vi "behavior_test_no_output.vi"() -> ()   [LabVIEW 2019]
doc: "The myRIO Project template acquires acceleration data from the onboard accelerometer and displays the changes of acceleration values in a waveform chart."
uses:
  <vilib>/myRIO/Common/Instrument Driver Framework/myRIO v1.0/Encoder/typedefs/Encoder Signal Mode.ctl
  <vilib>/myRIO/Instrument Drivers/Onboard IO/Encoder/typedefs/Encoder Reference.ctl
  <vilib>/myRIO/Common/Instrument Driver Framework/Utilities/typedefs/myRIO Generic Hardware Reference.ctl
  <vilib>/myRIO/Common/Instrument Driver Framework/Utilities/typedefs/Hardware Version Enum.ctl
  <vilib>/myRIO/Common/Instrument Driver Framework/Utilities/typedefs/myRIO v1.0 Reference.ctl
  <vilib>/myRIO/Common/Instrument Driver Framework/Utilities/typedefs/Generic FPGA Reference.ctl
  <vilib>/myRIO/Common/Instrument Driver Framework/myRIO v1.0/Encoder/typedefs/Encoder Channels Enum.ctl
  <vilib>/myRIO/Common/Instrument Driver Framework/myRIO v1.0/Encoder/typedefs/Encoder Configuration v1.0.ctl
  <vilib>/userdefined/High Color/nirio_resource_hc.ctl
  <vilib>/myRIO/Instrument Drivers/Onboard IO/DIO/typedefs/DIO Reference.ctl
  <vilib>/myRIO/Common/Instrument Driver Framework/myRIO v1.0/DIO/typedefs/DIO Channels List.ctl
  <vilib>/myRIO/Common/Instrument Driver Framework/myRIO v1.0/DIO/typedefs/DIO Channels Enum.ctl
  <vilib>/myRIO/Common/Instrument Driver Framework/Utilities/vis/Is FPGA Ref Available.vi
  <vilib>/myRIO/Common/Instrument Driver Framework/myRIO v1.0/Encoder/vis/myRIO v1.1 Open Encoder.vi
  <vilib>/myRIO/Instrument Drivers/Onboard IO/Encoder/vis/Read.vi
  <vilib>/myRIO/Common/Instrument Driver Framework/myRIO v1.0/DIO/vis/myRIO v1.1 Open DIO.vi
  <vilib>/myRIO/Instrument Drivers/Onboard IO/DIO/vis/Write.vi
  <vilib>/myRIO/Instrument Drivers/Onboard IO/DIO/vis/Read.vi
  <vilib>/myRIO/Common/Instrument Driver Framework/Utilities/vis/Validate Channels.vi
  <vilib>/myRIO/Common/Instrument Driver Framework/myRIO v1.0/Encoder/vis/myRIO v1.0 Reserve Encoder.vi
  <vilib>/myRIO/Common/Instrument Driver Framework/myRIO v1.0/DIO/vis/myRIO v1.0 Reserve DIO.vi
  <vilib>/myRIO/Common/Instrument Driver Framework/myRIO v1.0/Encoder/vis/myRIO v1.0 Build MUX Configuration Encoder.vi
  <vilib>/myRIO/Common/Instrument Driver Framework/myRIO v1.0/Resource Manager/vis/myRIO v1.0 Reserve Channel List.vi
  <vilib>/myRIO/Common/Instrument Driver Framework/myRIO v1.0/DIO/vis/myRIO v1.0 Build MUX Configuration DIO.vi
  <vilib>/myRIO/Common/Instrument Driver Framework/myRIO v1.0/Resource Manager/vis/myRIO v1.0 Create Configuration List.vi
  <vilib>/myRIO/Common/Instrument Driver Framework/myRIO v1.0/Resource Manager/vis/myRIO v1.0 Reserve Channel.vi
  <vilib>/myRIO/Common/Instrument Driver Framework/myRIO v1.0/Resource Manager/vis/myRIO v1.0 Unreserve Channel.vi
  <vilib>/myRIO/Common/Instrument Driver Framework/myRIO v1.0/Resource Manager/vis/myRIO v1.0 Build Mutex Name.vi
  <vilib>/Utility/VariantDataType/GetNumericInfo.vi
  <vilib>/Utility/error.llb/Error Cluster From Error Code.vi
  <vilib>/myRIO/Common/Instrument Driver Framework/myRIO v1.0/myRIO v1.1 Open.vi
  <vilib>/myRIO/Common/Instrument Driver Framework/Utilities/vis/IO Manager.vi
  <vilib>/myRIO/Common/Instrument Driver Framework/Utilities/vis/Configuration Manager.vi
  <vilib>/myRIO/Common/Instrument Driver Framework/myRIO v1.0/Resource Manager/vis/myRIO v1.0 Configure IO.vi
  <vilib>/myRIO/Common/Instrument Driver Framework/myRIO v1.0/myRIO v1.0 Close.vi
  <vilib>/myRIO/Common/Instrument Driver Framework/myRIO v1.0/Encoder/vis/myRIO v1.0 Configure Encoder.vi
  <vilib>/myRIO/Common/Instrument Driver Framework/myRIO v1.0/Encoder/vis/myRIO v1.0 Read Encoder.vi
  <vilib>/myRIO/Common/Instrument Driver Framework/myRIO v1.0/DIO/vis/myRIO v1.0 Read DIO.vi
  <vilib>/myRIO/Common/Instrument Driver Framework/myRIO v1.0/DIO/vis/myRIO v1.0 Write DIO.vi
  <vilib>/myRIO/Express VI/Onboard IO/Encoder/Encoder Express VI.xnode
  <vilib>/myRIO/Instrument Drivers/Onboard IO/Encoder/vis/myRIO Encoder Open.xnode
  <vilib>/myRIO/Common/Instrument Driver Framework/myRIO v1.0/Encoder/typedefs/Encoder Count Direction Enum.ctl
  <vilib>/myRIO/Express VI/Onboard IO/DI/DI Express VI.xnode
  <vilib>/myRIO/Instrument Drivers/Onboard IO/DIO/vis/myRIO DIO Open.xnode
  <vilib>/myRIO/Express VI/Onboard IO/DO/DO Express VI.xnode
  <vilib>/myRIO/Instrument Drivers/Onboard IO/Encoder/Encoder.lvlib
  <vilib>/myRIO/Instrument Drivers/Onboard IO/DIO/DIO.lvlib
panel:
  out "Reward_mat":dbl[](array[numeric])
  out "Reward":bool=TRUE
  out "Trial":u32
  out "Frame clock":i32
  out "Licks":u32
  out "Lick":bool
  out "Output":dbl[][](array[numeric])
  out "Time":dbl
  out "Overflow?":bool
  out "Counter Value":i32
  out "Velocity":dbl
  out "Velocity Plot":dbl[](graph)
  out "Velocity array":dbl[](array[numeric])
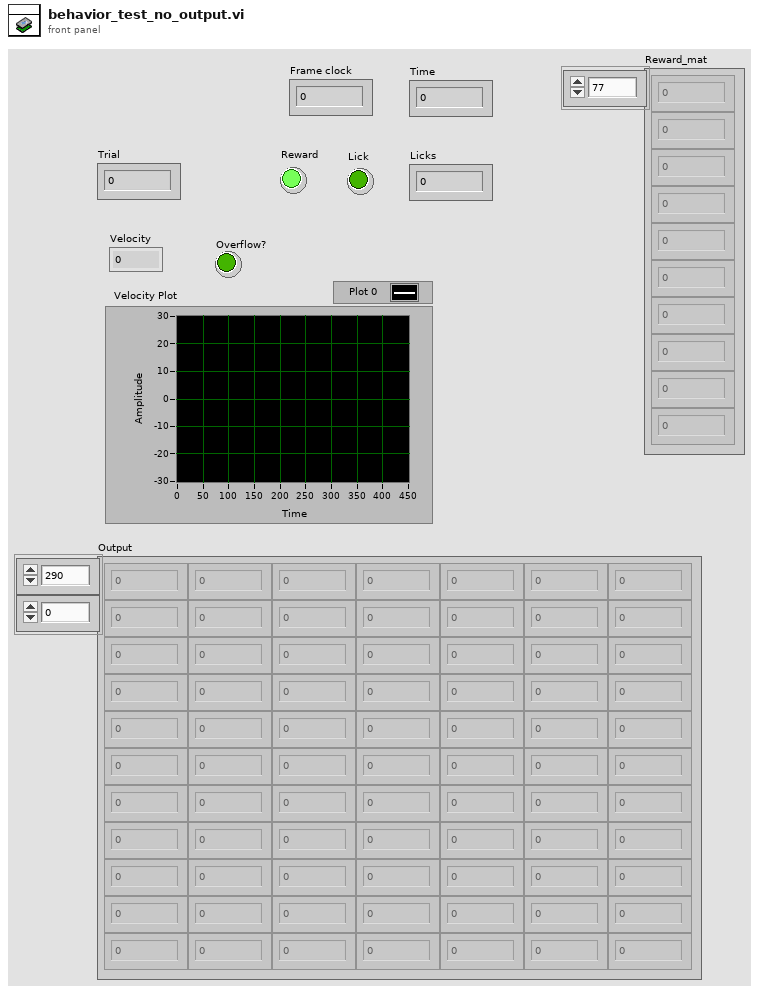
[diagram p1: front panel]
types:
  T1 = typedef "Encoder.lvlib/Encoder Reference.ctl" = cluster{"myRIO Reference":T2, "Encoder Channels Enum":T6}
  T2 = typedef "myRIO Generic Hardware Reference.ctl" = cluster{"myRIO Model":T3, "myRIO Hardware Reference":T4}
  T3 = typedef "Hardware Version Enum.ctl" = enum16{"Unknown", "myRIO-1900", "myRIO-1950", "roboRIO", "NI ELVIS RIO CM", "ELVIS III"}
  T4 = typedef "myRIO v1.0 Reference.ctl" = cluster{"Generic FPGA Reference":T5, "Allow multiple opens":bool}
  T5 = typedef "Generic FPGA Reference.ctl" = refnum<k20>
  T6 = typedef "Encoder Channels Enum.ctl" = enum16{"Not Connected", "C/ENC0", "C/ENC1", "A/ENC", "A/ENC0", "A/ENC1", "A/ENC2", "A/ENC3", "A/ENC4", "A/ENC5", "A/ENC6", "A/ENC7", "A/ENC8", "A/ENC9", "B/ENC", "B/ENC0", "B/ENC1", "B/ENC2", "B/ENC3", "B/ENC4", "B/ENC5", "B/ENC6", "B/ENC7", "B/ENC8", "B/ENC9", "DIO/ENC0", "DIO/ENC1", "DIO/ENC2", "DIO/ENC3", "DIO/ENC4"}
  T7 = typedef "Encoder Signal Mode.ctl" = enum16{"Quadrature phase signal", "Step and direction signal"}
  T8 = typedef "nirio_resource_hc.ctl" = tag
  T9 = typedef "DIO.lvlib/DIO Reference.ctl" = cluster{"myRIO Reference":T2, "DIO Channels List":T10}
  T10 = typedef "DIO Channels List.ctl" = T11[]
  T11 = typedef "DIO Channels Enum.ctl" = enum16{"Not Connected", "C/DIO0", "C/DIO1", "C/DIO2", "C/DIO3", "C/DIO4", "C/DIO5", "C/DIO6", "C/DIO7", "A/DIO0", "A/DIO1", "A/DIO2", "A/DIO3", "A/DIO4", "A/DIO5", "A/DIO6", "A/DIO7", "A/DIO8", "A/DIO9", "A/DIO10", "A/DIO11", "A/DIO12", "A/DIO13", "A/DIO14", "A/DIO15", "A/DIO16", "A/DIO17", "A/DIO18", "A/DIO19", "B/DIO0", "B/DIO1", "B/DIO2", "B/DIO3", "B/DIO4", "B/DIO5", "B/DIO6", "B/DIO7", "B/DIO8", "B/DIO9", "B/DIO10", "B/DIO11", "B/DIO12", "B/DIO13", "B/DIO14", "B/DIO15", "B/DIO16", "B/DIO17", "B/DIO18", "B/DIO19", "LED0", "LED1", "LED2", "LED3", "Button0", "DIO/DIO0", "DIO/DIO1", "DIO/DIO2", "DIO/DIO3", "DIO/DIO4", "DIO/DIO5", "DIO/DIO6", "DIO/DIO7", "DIO/DIO8", "DIO/DIO9", "SPI/CS0", "SPI/CS1", "SPI/CS2", "SPI/CS3", "LED RADIO (Green)", "LED RADIO (Red)", "LED COMM (Green)", "LED COMM (Red)", "LED MODE (Green)", "LED MODE (Red)"}
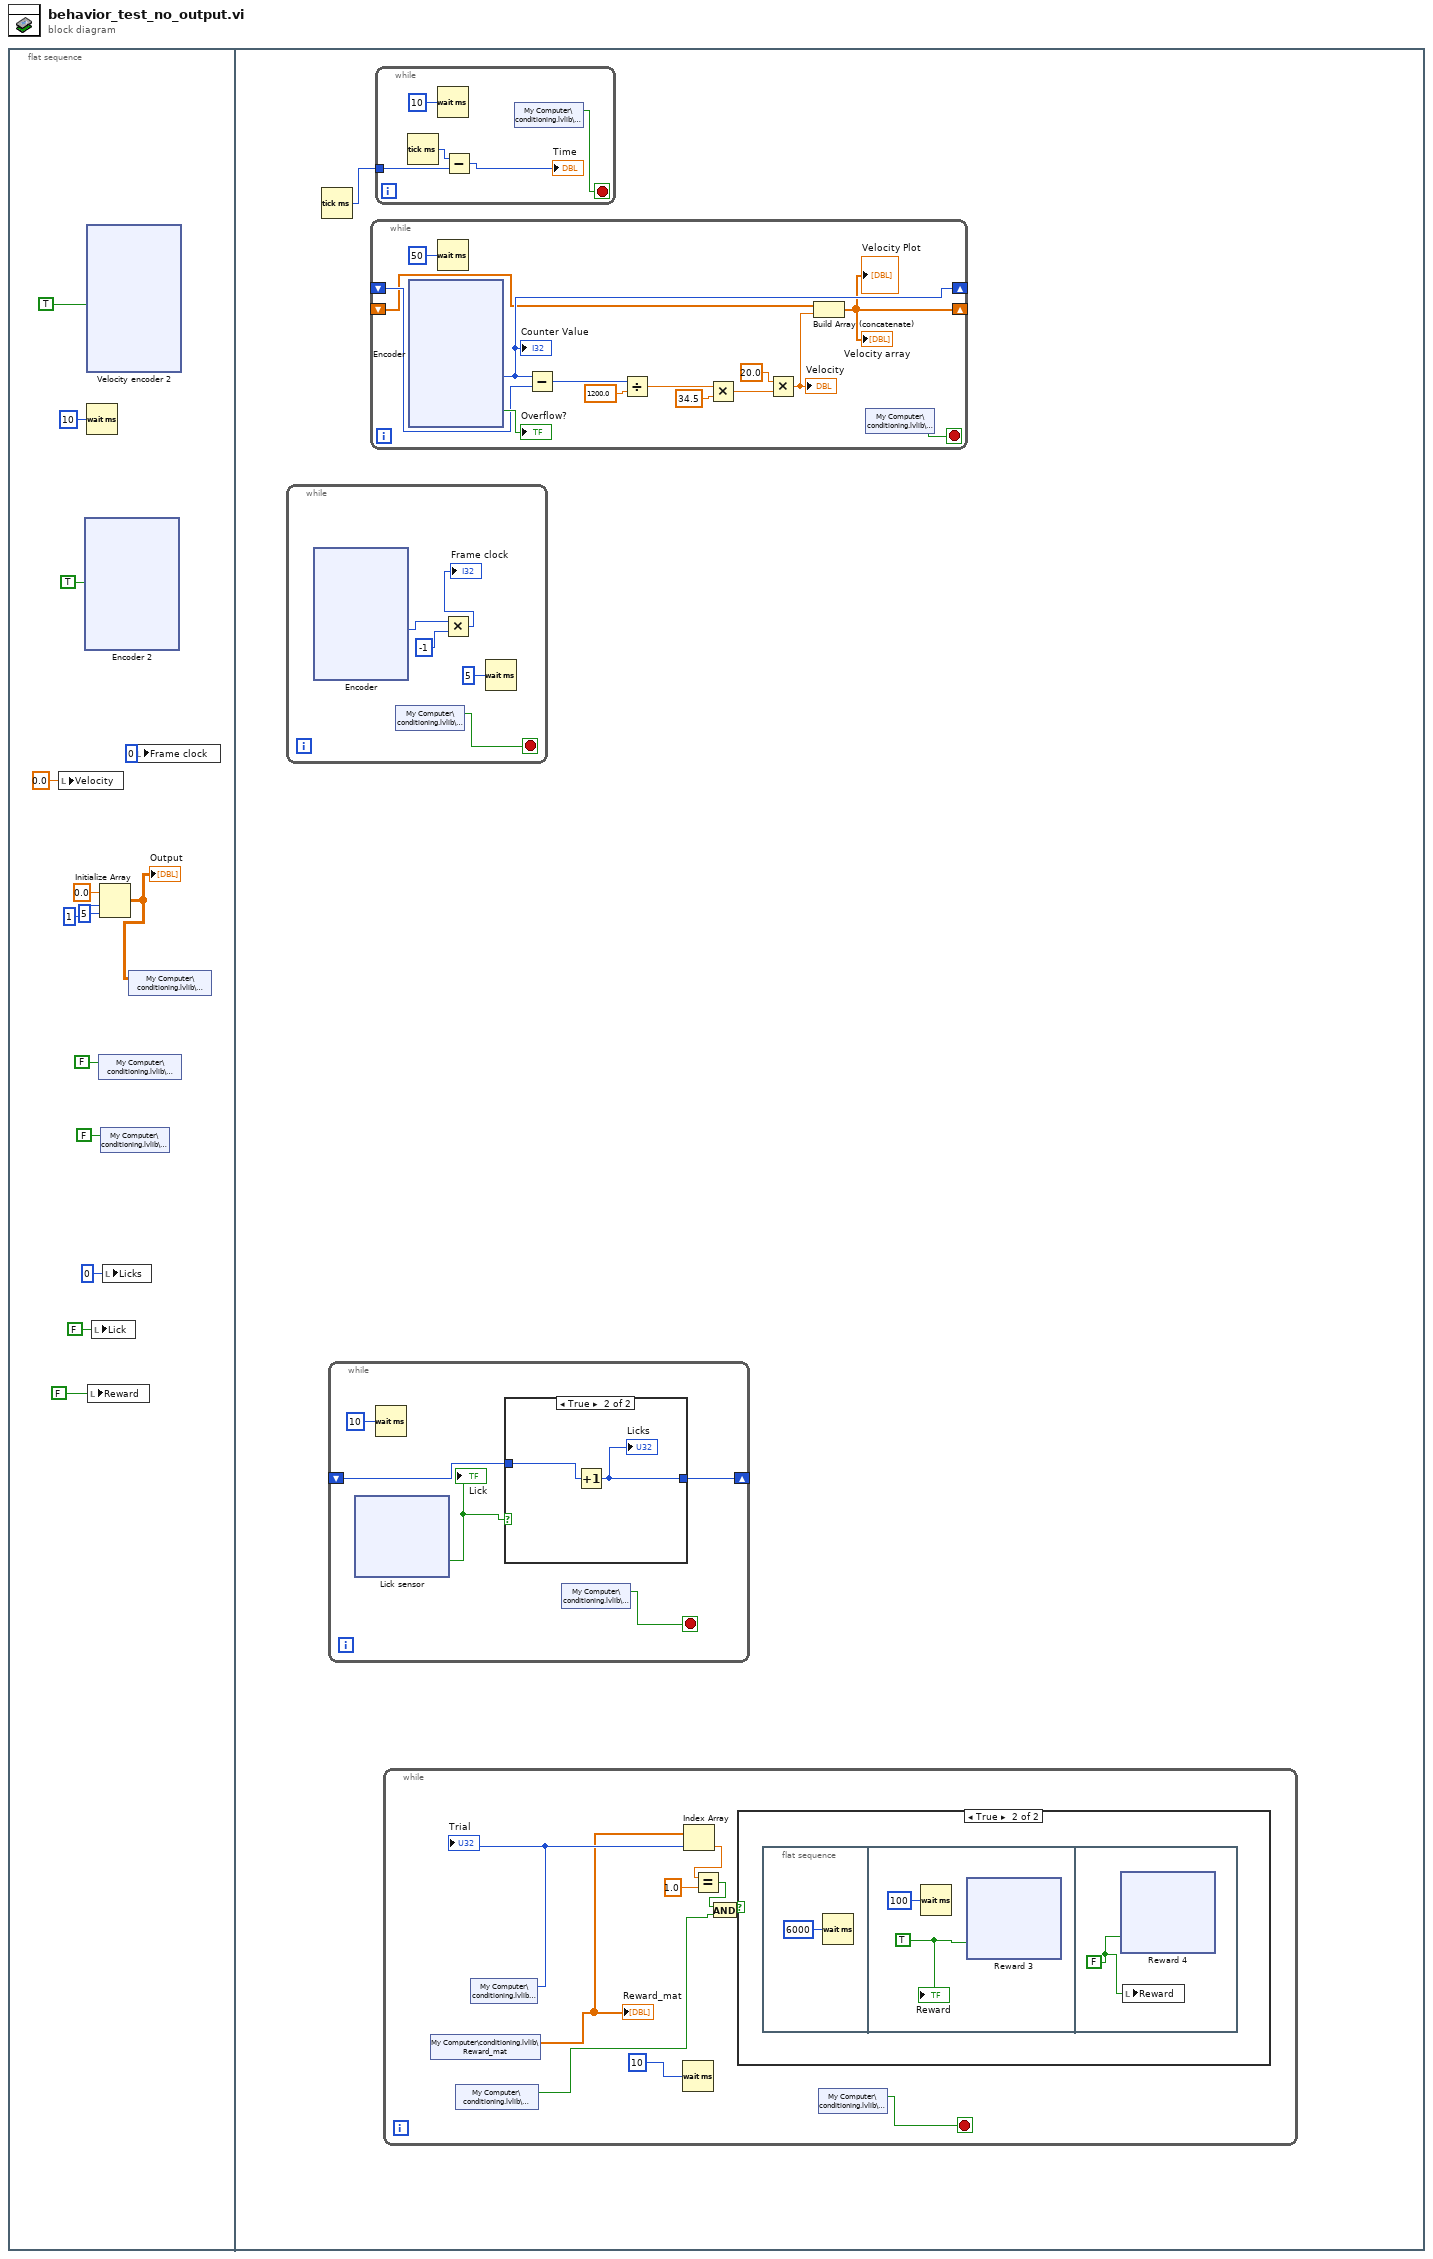
[diagram p0: block diagram]
diagram:
  n1 = flat-sequence {
    frame #0 {
      n2 = local write "Velocity"(0.0 ("Velocity")) -> ()
      n3 = xnode "Encoder 2"("Reset Counter"=TRUE) -> ()  [unwired: 1 in, 4 out]
      n4 = xnode "Velocity encoder 2"("Reset Counter"=TRUE) -> ()  [unwired: 1 in, 4 out]
      n5 = Wait (ms)(milliseconds to wait=u32 10) -> ()  [unwired: 1 out]
      n6 = local write "Reward"(FALSE ("Give reward")) -> ()
      n7 = local write "Lick"(FALSE ("Lick")) -> ()
      n8 = shared-variable "My Computer\\conditioning.lvlib\\Display"(FALSE ("Display")) -> ()  [unwired: 1 in, 1 out]
      n9 = Initialize Array(0.0 ("element"), 1 ("dimension size"), 5 ("dimension size")) -> (w8:dbl[][])
      "Output" <- w8
      n10 = shared-variable "My Computer\\conditioning.lvlib\\Stop"(FALSE ("Stop")) -> ()  [unwired: 1 in, 1 out]
      n11 = local write "Licks"(u32 0 ("Licks")) -> ()
      n12 = shared-variable "My Computer\\conditioning.lvlib\\Output"(w8) -> ()  [unwired: 1 in, 1 out]
      n13 = local write "Frame clock"(u32 0 ("Frames")) -> ()
    }
    frame #1 {
      n14 = while {
        stop <- w192 stop-if-true
        n15 = xnode "Encoder"() -> ("Counter Value"=w195:i32)  [unwired: 2 in, 3 out]
        n16 = shared-variable "My Computer\\conditioning.lvlib\\Stop"() -> (w192:bool)  [unwired: 1 in, 1 out]
        n17 = Multiply(x=w195, y=-1) -> (x*y=→"Frame clock":i32)
        n18 = Wait (ms)(milliseconds to wait=u32 5) -> ()  [unwired: 1 out]
      }
      n19 = Tick Count (ms)() -> (millisecond timer value=w107:u32)
      n20 = while {
        shift-right: [w243] -> _
        shift-left: _ -> [w242]
        stop <- w246 stop-if-true
        n21 = xnode "Lick sensor"() -> ("C/DIO1 (DIO1)"=w244:bool)  [unwired: 1 in, 1 out]
        "Lick" <- w244
        n22 = Wait (ms)(milliseconds to wait=u32 10) -> ()  [unwired: 1 out]
        n23 = case shown="True" w244 {
          tunnel: [w247 w249] -> w243
          tunnel: w242 -> [w247 w248]
          frame False {
          }
          frame True {
            n24 = Increment(x=w248) -> (x+1=w249:u32)
            "Licks" <- w249
          }
        }
        n25 = shared-variable "My Computer\\conditioning.lvlib\\Stop"() -> (w246:bool)  [unwired: 1 in, 1 out]
      }
      n26 = while {
        shift-right: [w295] -> _
        shift-left: _ -> [w296]
        shift-right: [w287] -> _
        shift-left: _ -> [w286]
        stop <- w285 stop-if-true
        n27 = xnode "Encoder"() -> ("Counter Value"=w295:i32, "Overflow?"=→"Overflow?":bool)  [unwired: 2 in, 2 out]
        "Counter Value" <- w295
        n28 = Wait (ms)(milliseconds to wait=u32 50) -> ()  [unwired: 1 out]
        n29 = Subtract(x=w295, y=w296) -> (x-y=w288:i32)
        n30 = Divide(x=w288, y=1200.0 ("600")) -> (x/y=w293:dbl)
        n31 = Multiply(x=w293, y=34.5) -> (x*y=w291:dbl)
        n32 = Multiply(x=20.0, y=w291) -> (x*y=w289:dbl)
        "Velocity" <- w289
        n33 = Build Array (concatenate)(w286, w289) -> (w287:dbl[])
        "Velocity Plot" <- w287
        "Velocity array" <- w287
        n34 = shared-variable "My Computer\\conditioning.lvlib\\Stop"() -> (w285:bool)  [unwired: 1 in, 1 out]
      }
      n35 = while {
        tunnel: w107 -> [w348]
        stop <- w346 stop-if-true
        n36 = Tick Count (ms)() -> (millisecond timer value=w349:u32)
        n37 = Wait (ms)(milliseconds to wait=u32 10) -> ()  [unwired: 1 out]
        n38 = Subtract(x=w349, y=w348) -> (x-y=→"Time":u32)
        n39 = shared-variable "My Computer\\conditioning.lvlib\\Stop"() -> (w346:bool)  [unwired: 1 in, 1 out]
      }
      n40 = while {
        stop <- w108 stop-if-true
        n41 = shared-variable "My Computer\\conditioning.lvlib\\Reward_mat"() -> (w114:dbl[])  [unwired: 1 in, 1 out]
        "Reward_mat" <- w114
        n42 = shared-variable "My Computer\\conditioning.lvlib\\Display"() -> (w110:bool)  [unwired: 1 in, 1 out]
        n43 = shared-variable "My Computer\\conditioning.lvlib\\Trial"() -> (w115:u32)  [unwired: 1 in, 1 out]
        "Trial" <- w115
        n44 = Wait (ms)(milliseconds to wait=u32 10) -> ()  [unwired: 1 out]
        n45 = Index Array(array=w114, index=w115) -> (element=w113:dbl)
        n46 = Equal?(x=w113, y=1.0) -> (x = y?=w111:bool)
        n47 = And(x=w111, y=w110) -> (x .and. y?=w109:bool)
        n48 = case shown="True" w109 {
          frame False {
          }
          frame True {
            n49 = flat-sequence {
              frame #0 {
                n50 = Wait (ms)(milliseconds to wait=u32 6000) -> ()  [unwired: 1 out]
              }
              frame #1 {
                w118 = TRUE ("C/DIO0 (DIO0)")
                n51 = Wait (ms)(milliseconds to wait=u32 100) -> ()  [unwired: 1 out]
                n52 = xnode "Reward 3"("C/DIO0 (DIO0)"=w118) -> ()  [unwired: 1 in, 1 out]
                "Reward" <- w118
              }
              frame #2 {
                w155 = FALSE ("C/DIO0 (DIO0)")
                n53 = xnode "Reward 4"("C/DIO0 (DIO0)"=w155) -> ()  [unwired: 1 in, 1 out]
                n54 = local write "Reward"(w155) -> ()
              }
            }
          }
        }
        n55 = shared-variable "My Computer\\conditioning.lvlib\\Stop"() -> (w108:bool)  [unwired: 1 in, 1 out]
      }
    }
  }
